vi "ti2_getXPos.vi"(8 "error in (no error)":errorcluster) -> (0 "error out":errorcluster, 3 "x Position (um)":dbl)   [LabVIEW 2018, in "ti2lv.lvlib"]
uses:
  ti2lv.lvlib
  ti2wrap/x64/Release/ti2wrap.dll
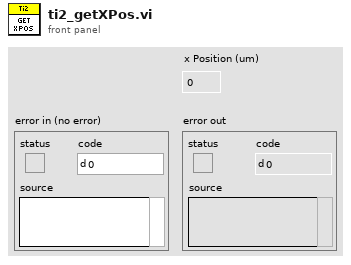
[diagram p1: front panel]
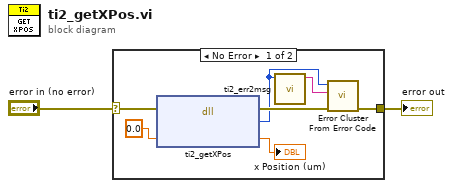
[diagram p0: block diagram]
diagram:
  n1 = case shown="No Error" "error in (no error)" {
    selector: "error in (no error)" -> [w8 w10]
    tunnel: [w9 w10] -> w1
    frame No Error {
      n2 = dll-call lib="C:/LVCUR/Flash Gordon v0.6.1b/Hardware/Ti2/ti2wrap/x64/Release/ti2wrap.dll" fn="ti2_getXPos"(error in=w8, "xPos_um"=0.0 ("filterPos")) -> (error out=w7:errorcluster, "return type"=w6:i32, "xPos_um"=→"x Position (um)":dbl)  [unwired: 2 in, 1 out]
      n3 = call "ti2_err2msg.vi"("Error Code"=w6) -> ("Error Message"=w5:string)  [unwired: 10 in]
      n4 = call <vilib>:"Error Cluster From Error Code.vi"("error in (no error)"=w7, "error message (\"\")"=w5, "error code (0)"=w6) -> ("error out"=w9:errorcluster)  [unwired: 6 in]
    }
    frame Error {
    }
  }
  "error out" <- w1
